vi "Sine_Wave_Generator.vi"() -> ()   [LabVIEW 2020]
uses:
  <vilib>/measure/NI_MABase.lvlib
panel:
  out "Waveform Graph subtract":waveform(dbl)(graph)
  out "Waveform Graph add":waveform(dbl)(graph)
  out "Waveform Graph squared":waveform(dbl)(graph)
  out "Waveform Graph":waveform(dbl)(graph)
  in  "Frequency":dbl(knob) scale=0.0..100.0
  in  "Amplitude":dbl(knob) scale=0.0..10.0
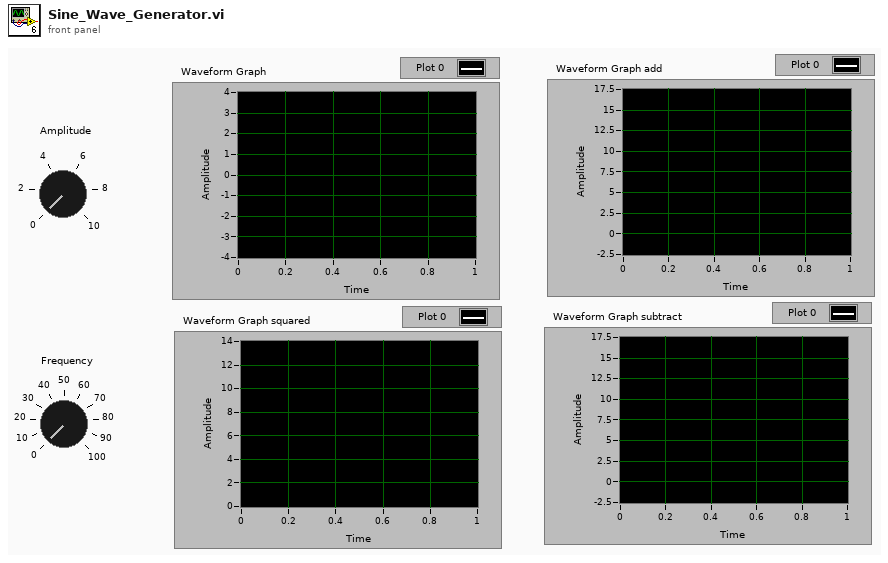
[diagram p1: front panel]
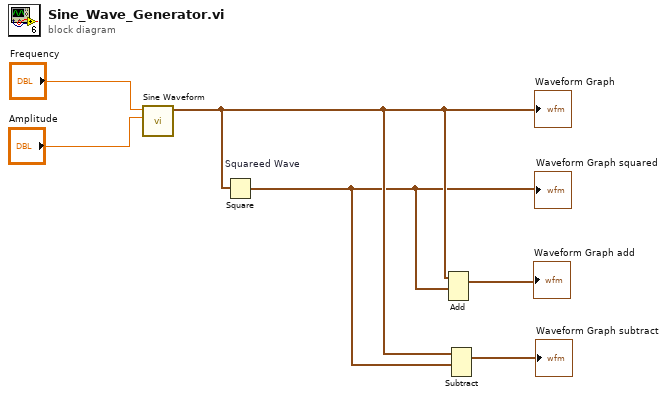
[diagram p0: block diagram]
diagram:
  n1 = call <vilib>:"Sine Waveform.vi"("amplitude"="Amplitude", "frequency"="Frequency") -> ("signal out"=w4:waveform(dbl))  [unwired: 8 in, 1 out]
  "Waveform Graph" <- w4
  n2 = Square "Squareed Wave"(x=w4) -> (x^2=w3:waveform(dbl))
  "Waveform Graph squared" <- w3
  n3 = Add(1:w3, 2:w4) -> (0:→"Waveform Graph add":waveform(dbl))  [unwired: 1 in, 1 out]
  n4 = Subtract(1:w3, 2:w4) -> (0:→"Waveform Graph subtract":waveform(dbl))  [unwired: 1 in, 1 out]
